vi "p2.vi"() -> ()   [LabVIEW 2021, in "d23.lvlib"]
uses:
  d23.lvlib
  AOC/AOC.lvlib
panel:
  in  "Example":string=".....\n..##.\n..#..\n.....\n..##.\n....."
  in  "Example":bool=TRUE
  out "Answer":i64
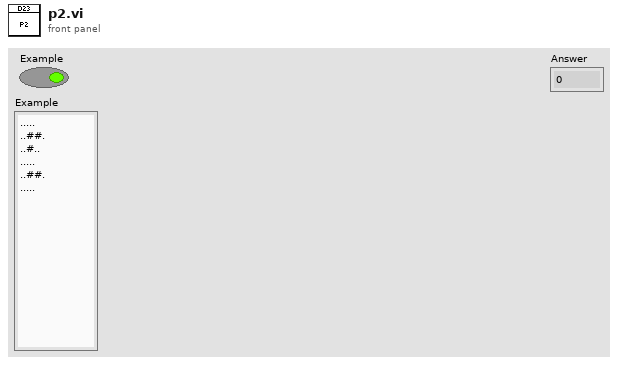
[diagram p1: front panel]
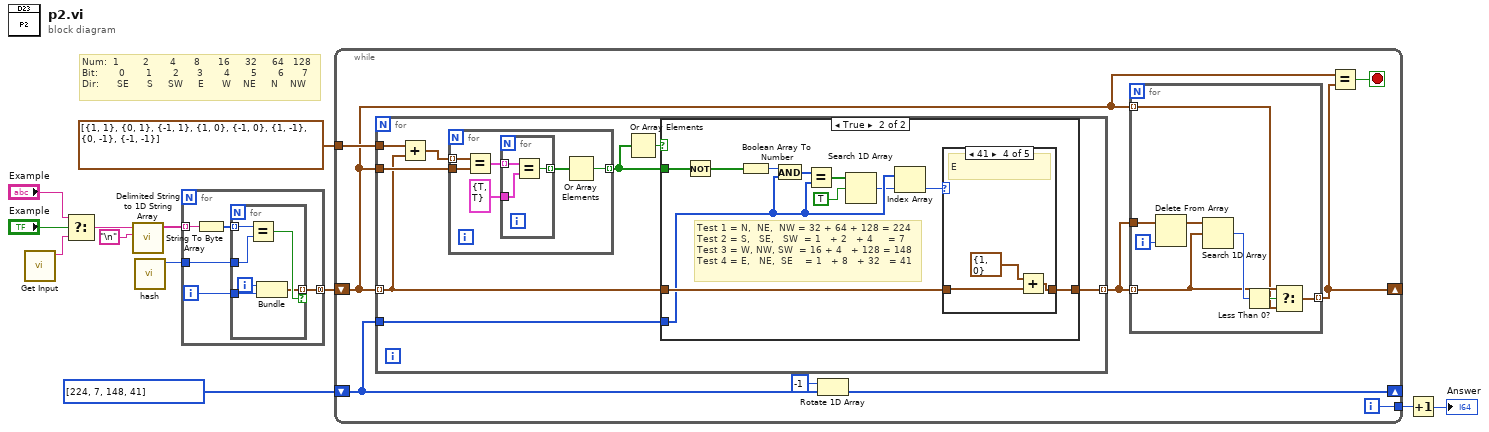
[diagram p0: block diagram]
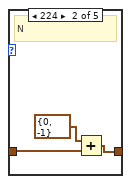
[diagram p4: hidden frame]
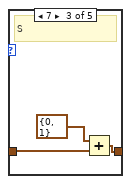
[diagram p5: hidden frame]
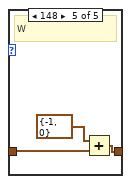
[diagram p6: hidden frame]
diagram:
  # "Num:  1        2       4      8      16     32     64   128\nBit:       0       1       2      3       4       5       6      7\nDir:      SE      S     SW     E      W    NE     N    NW"
  n1 = call "Get Input.vi"() -> ("Input"=w12:string)  [unwired: 11 in]
  n2 = Select(t="Example", s="Example", f=w12) -> (s? t:f=w11:string)
  n3 = call <vilib>:"Delimited String to 1D String Array.vi"("delimiter"="\n", "delimited string"=w11) -> ("string array"=w7:string[])  [unwired: 9 in]
  n4 = call "hash.vi"() -> ("#"=w6:u8)  [unwired: 11 in]
  n5 = for {
    tunnel: w7 -> [w17] mode=indexing
    tunnel: w6 -> [w15]
    tunnel: [w14] -> w5 mode=concatenating
    i -> [w13]
    n6 = String To Byte Array(string=w17) -> (unsigned byte array=w16:u8[])
    n7 = for {
      tunnel: w16 -> [w23] mode=indexing
      tunnel: w15 -> [w22]
      tunnel: [w20] -> w14 mode=indexing if=w21
      tunnel: w13 -> [w19]
      i -> [w18]
      n8 = Equal?(x=w23, y=w22) -> (x = y?=w21:bool)
      n9 = Bundle(w18, w19) -> (w20:cluster{i32, i32})  [unwired: 1 in]
    }
  }
  n10 = while {
    shift-right: [w26] -> _
    shift-left: w5 -> [w24]
    tunnel: cluster{i32, i32}[] [{1, 1}, {0, 1}, {-1, 1}, {1, 0}, {-1, 0}, {1, -1}, {0, -1}, {-1, -1}] -> [w32]
    shift-right: [w29] -> _
    shift-left: u8[] [224, 7, 148, 41] ("number") -> [w30]
    tunnel: [w25] -> w2
    i -> [w25]
    stop <- w27 stop-if-true
    n11 = for {
      tunnel: w24 -> [w44] mode=indexing
      tunnel: w24 -> [w47]
      tunnel: w32 -> [w45]
      tunnel: [w42] -> w31 mode=indexing
      tunnel: w30 -> [w41]
      n12 = Add(x=w45, y=w44) -> (x+y=w48:cluster{i32, i32}[])
      n13 = for {
        tunnel: w48 -> [w54] mode=indexing
        tunnel: w47 -> [w53]
        tunnel: [w49] -> w43 mode=indexing
        n14 = Equal?(x=w54, y=w53) -> (x = y?=w52:cluster{bool, bool}[])
        n15 = for {
          tunnel: w52 -> [w57] mode=indexing
          tunnel: cluster{bool, bool} {TRUE, TRUE} ("y") -> [w56]
          tunnel: [w55] -> w50 mode=indexing
          n16 = Equal?(x=w57, y=w56) -> (x = y?=w55:bool)
        }
        n17 = Or Array Elements(Boolean array=w50) -> (logical OR=w49:bool)
      }
      n18 = Or Array Elements(Boolean array=w43) -> (logical OR=w46:bool)
      n19 = case shown="True" w46 {
        tunnel: w44 -> [w58 w69]
        tunnel: [w58 w66] -> w42
        tunnel: w43 -> [_ w67]
        tunnel: w41 -> [_ w61]
        frame False {
        }
        frame True {
          # "Test 1 = N,  NE,  NW = 32 + 64 + 128 = 224\nTest 2 = S,   SE,   SW  = 1   + 2   + 4     = 7\nTest 3 = W, NW, SW  = 16 + 4   + 128 = 148\nTest 4 = E,   NE,  SE    = 1   + 8   + 32   = 41"
          n20 = Not(x=w67) -> (.not. x?=w65:bool[])
          n21 = Boolean Array To Number(Boolean array=w65) -> (number=w68:u8)
          n22 = And(x=w68, y=w61) -> (x .and. y?=w64:u8[])
          n23 = Equal?(x=w64, y=w61) -> (x = y?=w63:bool[])
          n24 = Search 1D Array(1D array=w63, element=TRUE) -> (index of element=w60:i32)  [unwired: 1 in]
          n25 = Index Array(array=w61, index=w60) -> (element=w59:u8)
          n26 = case shown="41" w59 {
            tunnel: w69 -> [w70 w72 w75 w78 w81]
            tunnel: [w70 w71 w74 w77 w80] -> w66
            frame Default {
              # "Can't Move"
            }
            frame 224 {
              # "N"
              n27 = Add(x=cluster{i32, i32} {0, -1}, y=w72) -> (x+y=w71:cluster{i32, i32})
            }
            frame 7 {
              # "S"
              n28 = Add(x=cluster{i32, i32} {0, 1}, y=w75) -> (x+y=w74:cluster{i32, i32})
            }
            frame 41 {
              # "E"
              n29 = Add(x=cluster{i32, i32} {1, 0}, y=w78) -> (x+y=w77:cluster{i32, i32})
            }
            frame 148 {
              # "W"
              n30 = Add(x=cluster{i32, i32} {-1, 0}, y=w81) -> (x+y=w80:cluster{i32, i32})
            }
          }
        }
      }
    }
    n31 = Rotate 1D Array(1:w30, 2:-1 ("n")) -> (0:w29:u8[])
    n32 = for {
      tunnel: w31 -> [w35] mode=indexing
      tunnel: w24 -> [w34] mode=indexing
      tunnel: w31 -> [w40]
      tunnel: [w33] -> w26 mode=indexing
      i -> [w39]
      n33 = Delete From Array(array=w40, index=w39) -> (array with subset deleted=w38:cluster{i32, i32}[])  [unwired: 1 in, 1 out]
      n34 = Search 1D Array(1D array=w38, element=w35) -> (index of element=w37:i32)  [unwired: 1 in]
      n35 = Less Than 0?(x=w37) -> (x < 0?=w36:bool)
      n36 = Select(t=w35, s=w36, f=w34) -> (s? t:f=w33:cluster{i32, i32})
    }
    n37 = Equal?(x=w24, y=w26) -> (x = y?=w27:bool)
  }
  n38 = Increment(x=w2) -> (x+1=→"Answer":i32)
